vi "Load_Database.vi"(8 "error in (no error)":errorcluster) -> (0 "error out":errorcluster, 3 "Database":T1[](array[typedef]))   [LabVIEW 2022 SP3]
uses:
  Database_element.ctl
  <vilib>/Utility/file.llb/Read Delimited Spreadsheet (string).vi
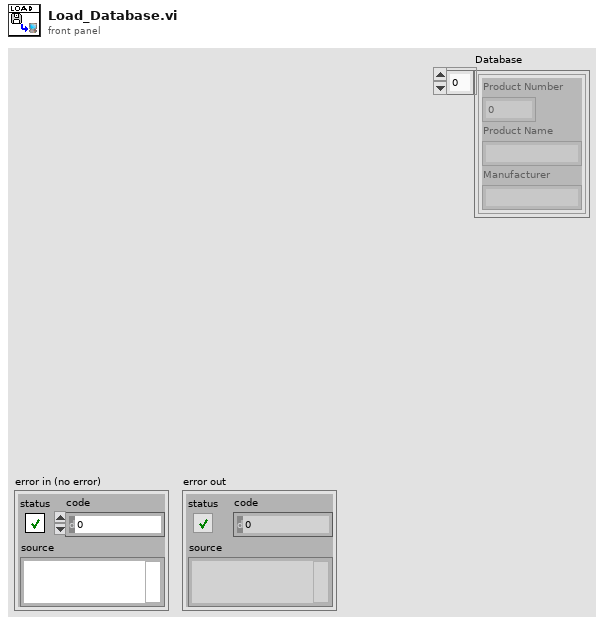
[diagram p1: front panel]
types:
  T1 = typedef "Database_element.ctl" = cluster{"Product Number":i32, "Product Name":string, "Manufacturer":string}
  T2 = enum16{"open", "replace", "create", "open or create", "replace or create", "replace or create with confirmation"}
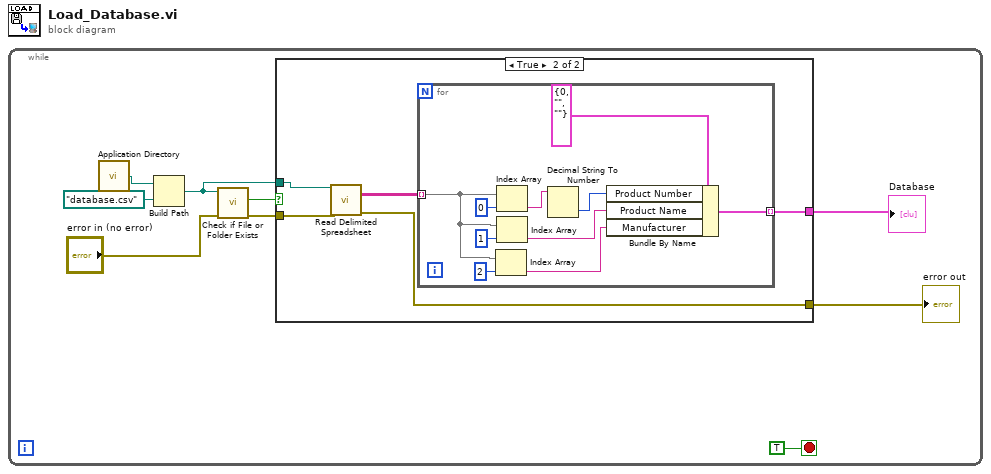
[diagram p0: block diagram]
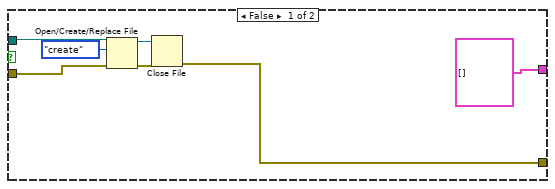
[diagram p2: hidden frame]
diagram:
  n1 = while {
    stop <- TRUE stop-if-true
    n2 = call <vilib>:"Application Directory.vi"() -> ("Application Directory"=w8:path)
    n3 = Build Path(base path=w8, name or relative path=path "database.csv") -> (appended path=w5:path)
    n4 = call <vilib>:"Check if File or Folder Exists.vi"("error in (no error)"="error in (no error)", "path"=w5) -> ("error out"=w3:errorcluster, "file or folder exists?"=w7:bool)  [unwired: 7 in, 1 out]
    n5 = case shown="True" w7 {
      tunnel: w5 -> [w16 w20]
      tunnel: w3 -> [w13 w19]
      tunnel: [w11 w17] -> w2
      tunnel: [T1[] [] w21] -> w1
      frame False {
        n6 = Open/Create/Replace File(file path (use dialog)=w16, error in=w13, operation (0:open)=T2."create") -> (refnum out=w14:refnum<file>, error out=w12:errorcluster)  [unwired: 3 in, 1 out]
        n7 = Close File(refnum=w14, error in=w12) -> (error out=w11:errorcluster)  [unwired: 1 out]
      }
      frame True {
        n8 = call-poly <vilib>:"Read Delimited Spreadsheet.vi"("file path (dialog if empty)"=w20, "error in (no error)"=w19) -> ("all rows"=w18:string[][], "error out"=w17:errorcluster)  [unwired: 8 in, 4 out]
        n9 = for {
          tunnel: [w30] -> w21 mode=indexing
          tunnel: w18 -> [w26] mode=indexing
          n10 = Index Array(array=w26, index=2) -> (element=w24:string)
          n11 = Index Array(array=w26, index=0) -> (element=w23:string)
          n12 = Index Array(array=w26, index=1) -> (element=w25:string)
          n13 = Decimal String To Number(string=w23) -> (number=w22:i32)  [unwired: 2 in, 1 out]
          n14 = Bundle By Name(cluster=T1 {"Product Number"=0, "Product Name"="", "Manufacturer"=""} ("Cluster"), "Product Number"=w22, "Product Name"=w25, "Manufacturer"=w24) -> (w30:T1)
        }
      }
    }
    "error out" <- w2
    "Database" <- w1
  }
